vi "DataPacker_SetAndGetMaxEventSize.vi"(8 "error in (no error)":errorcluster, 10 "Set Event Max Size":u32, 11 "DataPacker in":refnum<class "DataPacker.lvclass">) -> (0 "error out":errorcluster, 3 "DataPacker out":refnum<class "DataPacker.lvclass">)   [LabVIEW 2018, in "feGEM DataPacker.lvlib" / "DataPacker.lvclass"]
uses:
  DataPacker.lvclass
  DataPacker.lvclass/DataPacker.ctl
  DataStructures/GEM_BANK_CLUSTER_typedef.ctl
  DataStructures/GEM_DATA_cluster_typedef.ctl
  463ee4ca-1a32-4bcd-a49a-e30ed6d1892b.vi
  da89cbaf-4c68-4093-8bad-7eae00197743.vi
  feGEM DataPacker.lvlib
  DataStructures/GEM_BANK_ARRAY.lvclass
  <vilib>/Utility/SystemLogging/NI_SystemLogging.lvlib
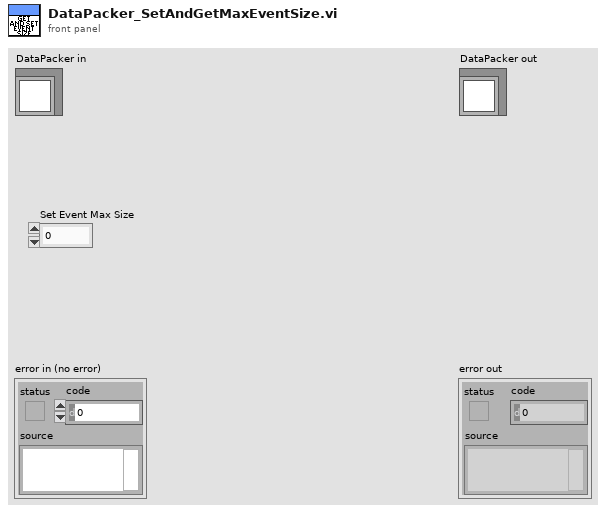
[diagram p1: front panel]
types:
  T1 = typedef "feGEM DataPacker.lvlib/GEM_BANK_CLUSTER_typedef.ctl" = cluster{"Category":string, "Variable Name":string, "Equipment description":string, "History Settings":u16, "Period to update history plots":u16, "GEM_DATA Cluster":T2}
  T2 = typedef "feGEM DataPacker.lvlib/GEM_DATA_cluster_typedef.ctl" = cluster{"DataType":string, "Formatted Data":u8[], "data byte order (Little Endian prefered)":enum16{"big-endian, network order", "native, host order", "little-endian"}}
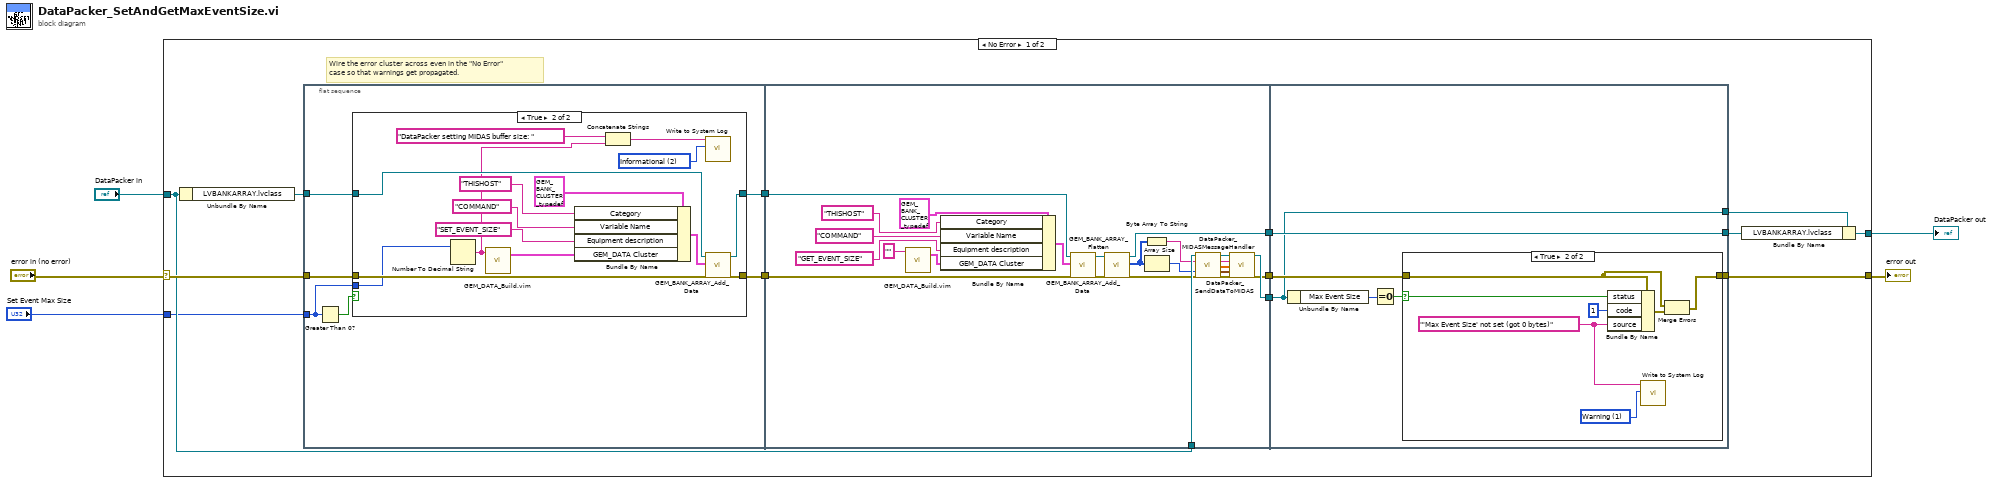
[diagram p0: block diagram]
diagram:
  n1 = case shown="No Error" "error in (no error)" {
    selector: "error in (no error)" -> [w13 w81]
    tunnel: [w12 w81] -> w4
    tunnel: [w7 w80] -> w2
    tunnel: "DataPacker in" -> [w10 w80]
    tunnel: "Set Event Max Size" -> [w6 _]
    frame No Error {
      # "Wire the error cluster across even in the \"No Error\"\ncase so that warnings get propagated."
      n2 = Unbundle By Name(w10) -> ("LVBANKARRAY.lvclass"=w14:refnum<class "GEM_BANK_ARRAY.lvclass">)
      n3 = flat-sequence {
        tunnel: [w22] -> w18
        tunnel: [w23] -> w17
        tunnel: w6 -> [w21]
        tunnel: w14 -> [w20]
        tunnel: w13 -> [w19]
        tunnel: [w53] -> w16
        tunnel: w18 -> [w63]
        tunnel: w17 -> [w64]
        tunnel: [w65] -> w15
        tunnel: w10 -> [w59]
        tunnel: [w54] -> w9
        tunnel: [w71] -> w12
        tunnel: w16 -> [w70]
        tunnel: w15 -> [w69]
        tunnel: [w69] -> w11
        tunnel: [w67] -> w8
        tunnel: w9 -> [w67]
        frame #0 {
          n4 = Greater Than 0?(x=w21) -> (x > 0?=w24:bool)
          n5 = case shown="True" w24 {
            tunnel: w20 -> [w26 w41]
            tunnel: [w26 w40] -> w23
            tunnel: w19 -> [w25 w39]
            tunnel: [w25 w38] -> w22
            tunnel: w21 -> [_ w37]
            frame False {
            }
            frame True {
              w28 = 2 items=["Error", "Warning", "Informational"] ("severity")
              n6 = Number To Decimal String(number=w37) -> (decimal integer string=w27:string)  [unwired: 1 in]
              n7 = call "GEM_DATA_Build.vim"("Any array in"=w27) -> ("GEM_BANK Cluster"=w32:T2)  [unwired: 2 in, 1 out]
              n8 = Bundle By Name(cluster=T1 {"Category"="", "Variable Name"="", "Equipment description"="", "History Settings"=0, "Period to update history plots"=0, "GEM_DATA Cluster"={"DataType"="", "Formatted Data"=[], "data byte order (Little Endian prefered)"=enum."big-endian, network order"}} ("output cluster"), "Category"="THISHOST", "Variable Name"="COMMAND" ("data"), "Equipment description"="SET_EVENT_SIZE", "GEM_DATA Cluster"=w32) -> (w34:T1)
              n9 = Concatenate Strings("DataPacker setting MIDAS buffer size: " ("message"), w27) -> (w29:string)
              n10 = call <vilib>:"Write to System Log.vi"("severity"=w28, "message"=w29) -> ()  [unwired: 9 in, 1 out]
              n11 = call "GEM_BANK_ARRAY_Add_Data.vi"("error in (no error)"=w39, "GEM BANK Cluster"=w34, "LVBANKARRAY in"=w41) -> ("error out"=w38:errorcluster, "LVBANKARRAY out"=w40:refnum<class "GEM_BANK_ARRAY.lvclass">)  [unwired: 7 in]
            }
          }
        }
        frame #1 {
          n12 = call "GEM_DATA_Build.vim"("Any array in"="") -> ("GEM_BANK Cluster"=w44:T2)  [unwired: 2 in, 1 out]
          n13 = Bundle By Name(cluster=T1 {"Category"="", "Variable Name"="", "Equipment description"="", "History Settings"=0, "Period to update history plots"=0, "GEM_DATA Cluster"={"DataType"="", "Formatted Data"=[], "data byte order (Little Endian prefered)"=enum."big-endian, network order"}} ("output cluster"), "Category"="THISHOST", "Variable Name"="COMMAND", "Equipment description"="GET_EVENT_SIZE" ("data"), "GEM_DATA Cluster"=w44) -> (w60:T1)
          n14 = call "GEM_BANK_ARRAY_Add_Data.vi"("error in (no error)"=w63, "GEM BANK Cluster"=w60, "LVBANKARRAY in"=w64) -> ("error out"=w45:errorcluster, "LVBANKARRAY out"=w46:refnum<class "GEM_BANK_ARRAY.lvclass">)  [unwired: 7 in]
          n15 = call "GEM_BANK_ARRAY_Flatten.vi"("error in (no error)"=w45, "LVBANKARRAY in"=w46) -> ("error out"=w57:errorcluster, "Array"=w51:u8[], "LVBANKARRAY out"=w65:refnum<class "GEM_BANK_ARRAY.lvclass">)  [unwired: 7 in]
          n16 = Byte Array To String(unsigned byte array=w51) -> (string=w58:string)
          n17 = Array Size(array=w51) -> (size(s)=w50:i32)
          n18 = call "DataPacker_SendDataToMIDAS.vi"("DataPacker in"=w59, "data in"=w58, "data in length"=w50, "error in (no error)"=w57) -> ("DataPacker out"=w55:refnum<class "DataPacker.lvclass">, "MIDAS Reply"=w56:string, "Send Time, Recieve Time"=w49:dbl[], "MIDAS Comm finished"=w48:timestamp, "error out"=w52:errorcluster)  [unwired: 7 in]
          n19 = call "DataPacker_MIDASMessageHandler.vi"("DataPacker in"=w55, "Message"=w56, "Array"=w49, "MIDAS Comm finish time"=w48, "error in (no error)"=w52) -> ("DataPacker out"=w54:refnum<class "DataPacker.lvclass">, "error out"=w53:errorcluster)  [unwired: 9 in]
        }
        frame #2 {
          n20 = Unbundle By Name(w67) -> ("Max Event Size"=w66:u32)
          n21 = Equal To 0?(x=w66) -> (x = 0?=w68:bool)
          n22 = case shown="True" w68 {
            selector: w68 -> [_ w78]
            tunnel: w70 -> [w72 w77]
            tunnel: [w72 w75] -> w71
            frame False {
            }
            frame True {
              w73 = 1 items=["Error", "Warning", "Informational"] ("severity")
              w74 = "'Max Event Size' not set (got 0 bytes)" ("error source (\" \")")
              n23 = Bundle By Name(cluster=w77, "status"=w78, "code"=1 ("error code (no error:0)"), "source"=w74) -> (w76:errorcluster)
              n24 = call <vilib>:"Write to System Log.vi"("severity"=w73, "message"=w74) -> ()  [unwired: 9 in, 1 out]
              n25 = Merge Errors(w77, w76) -> (w75:errorcluster)
            }
          }
        }
      }
      n26 = Bundle By Name(cluster=w8, "LVBANKARRAY.lvclass"=w11) -> (w7:refnum<class "DataPacker.lvclass">)
    }
    frame Error {
    }
  }
  "error out" <- w4
  "DataPacker out" <- w2
